vi "Recoverable Errors.vi"() -> ()   [LabVIEW 2018]
uses:
  api/Failure Information.ctl
  api/Log Record.ctl
  api/logger_class/Internal Log Levels.ctl
  api/Log Levels.ctl
  api/configuration/handlers/file_handler/File Handler.lvclass
  C:/Users/Colin/Documents/software_projects/glog/src/api/extension/formatting_handler_interface/Formatting Handler.lvclass
  custom_classes/test_handler/Test Handler.lvclass
  <vilib>/ErrorRing/Error Ring.xnode
  api/logger_class/Logger.lvclass
  api/GLog.lvlib
  <vilib>/addons/_JKI.lib/Serialization/JSON/JKI JSON Serialization.lvlib
panel:
  out "failure info":T1 {"Log Record"."timestamp" format="%<%x %.3X>T"}
  out "error out":errorcluster
  out "result":bool
  # "Locals"
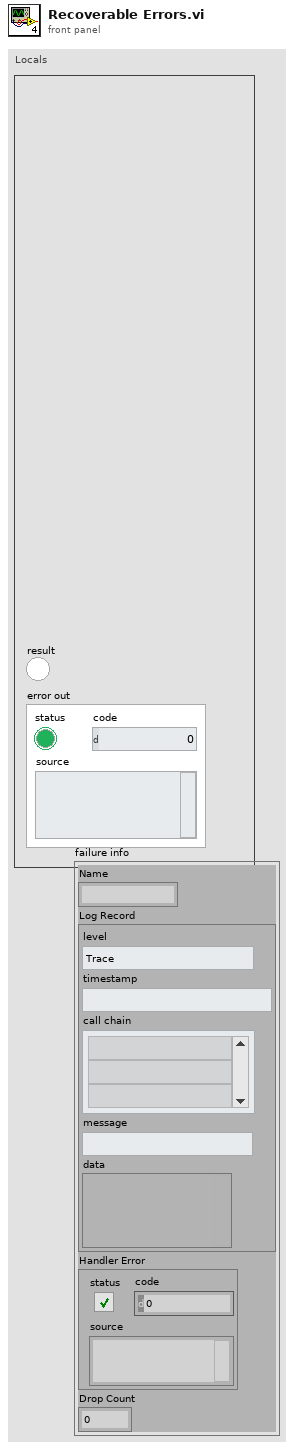
[diagram p1: front panel]
types:
  T1 = typedef "GLog.lvlib/Failure Information.ctl" = cluster{"Name":string, "Log Record":T2, "Handler Error":errorcluster, "Drop Count":u32}
  T2 = typedef "GLog.lvlib/Log Record.ctl" = cluster{"level":T3, "timestamp":timestamp, "call chain":string[], "message":string, "data":variant}
  T3 = typedef "GLog.lvlib/Internal Log Levels.ctl" = enum16{"Trace", "Debug", "Info", "Warning", "Error", "Critical", "Internal"}
  T4 = typedef "GLog.lvlib/Log Levels.ctl" = enum16{"Trace", "Debug", "Info", "Warning", "Error", "Critical"}
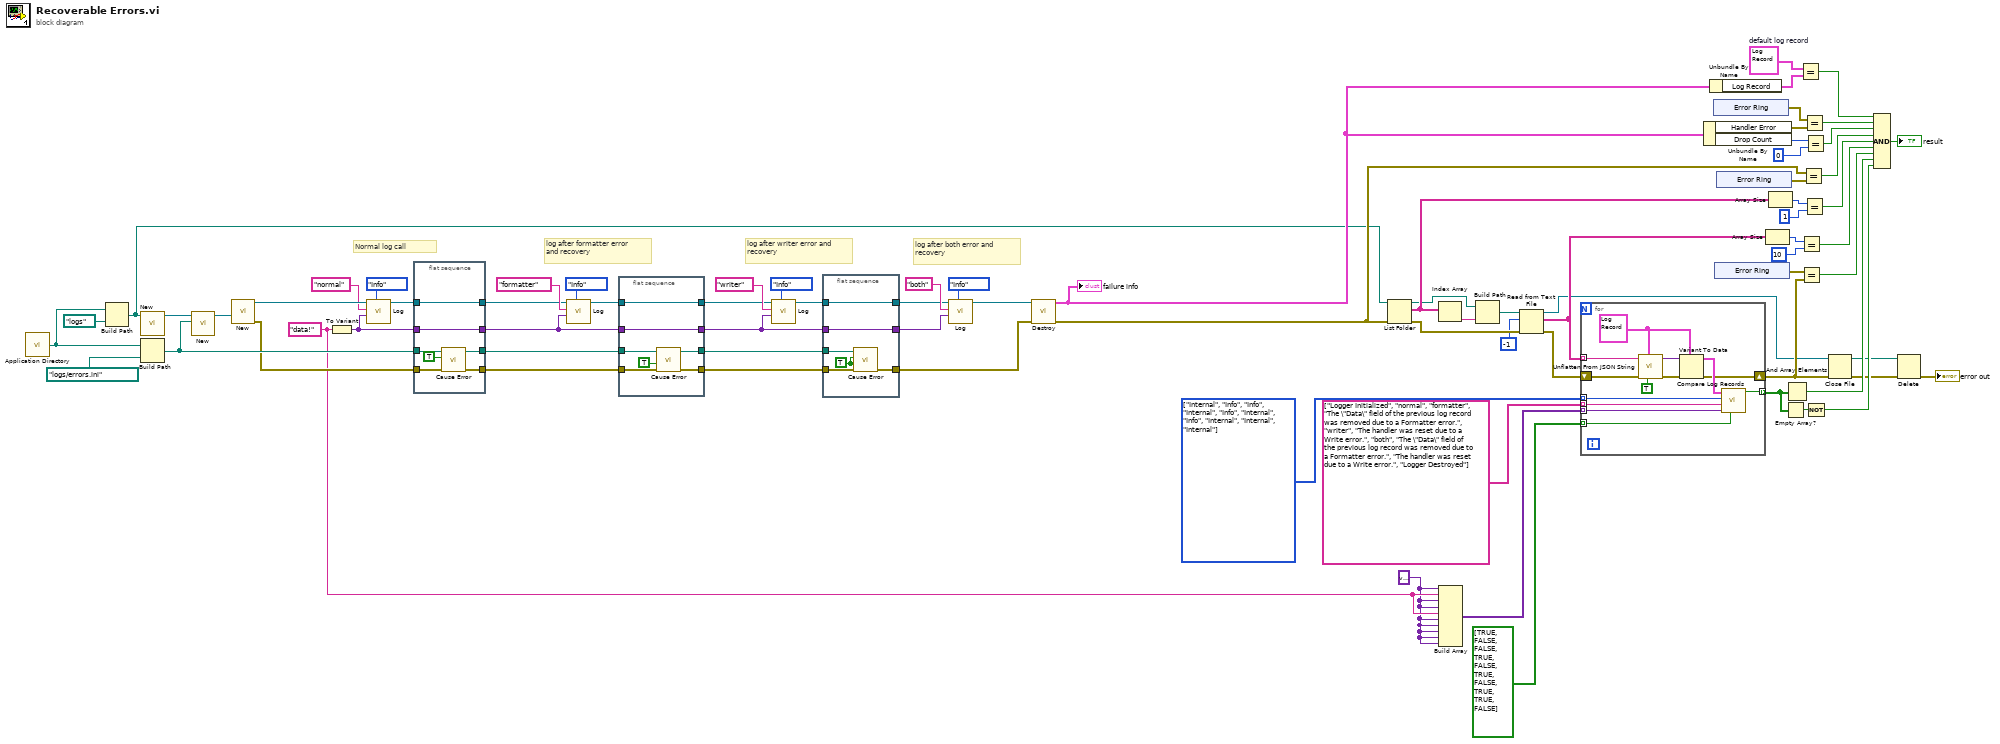
[diagram p0: block diagram]
diagram:
  w2 = variant
  w18 = T3[] [enum."Internal", enum."Info", enum."Info", enum."Internal", enum."Info", enum."Internal", enum."Info", enum."Internal", enum."Internal", enum."Internal"] items=["Trace", "Debug", "Info", "Warning", "Error", "Critical", "Internal"] ("expected log level")
  w38 = T2 {"level"=enum."Trace", "timestamp"=timestamp(0 s since 1904-01-01), "call chain"=[], "message"="", "data"=variant}  # default log record
  w15 = "data!" ("message")
  # "log after both error and recovery"
  # "log after writer error and recovery"
  # "log after formatter error and recovery"
  # "Normal log call"
  n1 = call <vilib>:"Application Directory.vi"() -> ("Application Directory"=w36:path)
  n2 = Build Path(base path=w36, name or relative path=path "logs") -> (appended path=w33:path)
  n3 = call "New.vi"("log directory (<app dir>/logs)"=w33) -> ("file handler"=w78:refnum<class "File Handler.lvclass">)  [unwired: 10 in]
  n4 = Build Path(base path=w36, name or relative path=path "logs/errors.ini") -> (appended path=w66:path)
  n5 = call "New.vi"("config file"=w66, "subhandler"=w78) -> ("test handler out"=w77:refnum<class "Test Handler.lvclass">)  [unwired: 9 in]
  n6 = call "New.vi"("log handler (file handler)"=w77) -> ("error out"=w65:errorcluster, "logger"=w75:refnum<class "Logger.lvclass">)  [unwired: 9 in]
  n7 = To Variant(anything=w15) -> (Variant=w52:variant)
  n8 = call "Log.vi"("log level"=Log_Levels."Info" ("level"), "data (null)"=w52, "message"="normal", "logger in"=w75) -> ("logger out"=w59:refnum<class "Logger.lvclass">)  [unwired: 7 in]
  n9 = flat-sequence {
    tunnel: w66 -> [w85]
    tunnel: w65 -> [w84]
    tunnel: [w83] -> w64
    tunnel: [w82] -> w63
    tunnel: [w80] -> w60
    tunnel: w59 -> [w80]
    tunnel: [w79] -> w51
    tunnel: w52 -> [w79]
    frame #0 {
      n10 = call "Cause Error.vi"("error in (no error)"=w84, "formatter error? (F)"=TRUE, "ini file path"=w85) -> ("error out"=w83:errorcluster, "ini file path"=w82:path)  [unwired: 7 in]
    }
  }
  n11 = call "Log.vi"("log level"=Log_Levels."Info" ("level"), "data (null)"=w51, "message"="formatter", "logger in"=w60) -> ("logger out"=w57:refnum<class "Logger.lvclass">)  [unwired: 7 in]
  n12 = flat-sequence {
    tunnel: w64 -> [w92]
    tunnel: w63 -> [w91]
    tunnel: [w89] -> w62
    tunnel: [w88] -> w61
    tunnel: [w87] -> w58
    tunnel: w57 -> [w87]
    tunnel: [w86] -> w49
    tunnel: w51 -> [w86]
    frame #0 {
      n13 = call "Cause Error.vi"("error in (no error)"=w92, "writer error? (F)"=TRUE, "ini file path"=w91) -> ("error out"=w88:errorcluster, "ini file path"=w89:path)  [unwired: 7 in]
    }
  }
  n14 = call "Log.vi"("log level"=Log_Levels."Info" ("level"), "data (null)"=w49, "message"="writer", "logger in"=w58) -> ("logger out"=w55:refnum<class "Logger.lvclass">)  [unwired: 7 in]
  n15 = flat-sequence {
    tunnel: w62 -> [w97]
    tunnel: w61 -> [w96]
    tunnel: [w95] -> w56
    tunnel: w55 -> [w95]
    tunnel: [w94] -> w53
    tunnel: [w93] -> w50
    tunnel: w49 -> [w93]
    frame #0 {
      w98 = TRUE ("writer error? (F)")
      n16 = call "Cause Error.vi"("error in (no error)"=w96, "writer error? (F)"=w98, "formatter error? (F)"=w98, "ini file path"=w97) -> ("error out"=w94:errorcluster)  [unwired: 6 in, 1 out]
    }
  }
  n17 = call "Log.vi"("log level"=Log_Levels."Info" ("level"), "data (null)"=w50, "message"="both", "logger in"=w56) -> ("logger out"=w54:refnum<class "Logger.lvclass">)  [unwired: 7 in]
  n18 = call "Destroy.vi"("error in (no error)"=w53, "logger in"=w54) -> ("error out"=w34:errorcluster, "failure info"=w40:T1)  [unwired: 8 in]
  "failure info" <- w40
  n19 = List Folder(path=w33, error in=w34) -> (path out=w27:path, filenames=w29:string[], error out=w25:errorcluster)  [unwired: 2 in, 1 out]
  n20 = Index Array(array=w29) -> (element=w28:string)  [unwired: 1 in]
  n21 = Build Array(w2, w15, w2, w2, w15, w2, w2, w2, w2, w2) -> (w16:variant[])
  n22 = Build Path(base path=w27, name or relative path=w28) -> (appended path=w26:path)
  n23 = Read from Text File(file (use dialog)=w26, count=-1, error in=w25) -> (refnum out=w6:refnum<file>, text=w20:string[], error out=w19:errorcluster)  [unwired: 1 in, 1 out]
  n24 = for {
    tunnel: w20 -> [w111] mode=indexing
    shift-right: [w106] -> w7
    shift-left: w19 -> [w108]
    tunnel: w18 -> [w105] mode=indexing
    tunnel: string[] ["Logger Initialized", "normal", "formatter", "The \"Data\" field of the previous log record was removed due to a Formatter error.", "writer", "The handler was reset due to a Write error.", "both", "The \"Data\" field of the previous log record was removed due to a Formatter error.", "The handler was reset due to a Write error.", "Logger Destroyed"] ("expected message") -> [w104] mode=indexing
    tunnel: w16 -> [w103] mode=indexing
    tunnel: bool[] [TRUE, FALSE, FALSE, TRUE, FALSE, TRUE, FALSE, TRUE, TRUE, FALSE] ("appended array") -> [w102] mode=indexing
    tunnel: [w101] -> w13 mode=indexing
    w100 = T2 {"level"=enum."Trace", "timestamp"=timestamp(0 s since 1904-01-01), "call chain"=[], "message"="", "data"=variant} ("default log record")
    n25 = call <vilib>:"Unflatten From JSON String.vi"("Nulls as Defaults (F)"=TRUE, "Type and Defaults"=w100, "error in (no error)"=w108, "JSON String"=w111) -> ("error out"=w110:errorcluster, "Variant"=w109:variant)  [unwired: 6 in]
    n26 = Variant To Data(error in=w110, type=w100, Variant=w109) -> (data=w107:T2, error out=w106:errorcluster)
    n27 = call "Compare Log Records.vi"("ignore data? (F)"=w102, "expected data"=w103, "expected message"=w104, "expected log level"=w105, "log record"=w107) -> ("match?"=w101:bool)  [unwired: 6 in]
  }
  n28 = Unbundle By Name(w40) -> ("Handler Error"=w48:errorcluster, "Drop Count"=w46:u32)
  n29 = Unbundle By Name(w40) -> ("Log Record"=w39:T2)
  n30 = xnode "Error Ring"() -> ("error out"=w47:errorcluster)
  n31 = xnode "Error Ring"() -> ("error out"=w14:errorcluster)
  n32 = xnode "Error Ring"() -> ("error out"=w44:errorcluster)
  n33 = Array Size(array=w20) -> (size(s)=w22:i32)
  n34 = Array Size(array=w29) -> (size(s)=w32:i32)
  n35 = Empty Array?(array=w13) -> (empty?=w12:bool)
  n36 = And Array Elements(Boolean array=w13) -> (logical AND=w10:bool)
  n37 = Equal?(x=w38, y=w39) -> (x = y?=w37:bool)
  n38 = Equal?(x=w22, y=10) -> (x = y?=w21:bool)
  n39 = Equal?(x=w14, y=w7) -> (x = y?=w11:bool)
  n40 = Equal?(x=w34, y=w44) -> (x = y?=w41:bool)
  n41 = Equal?(x=w47, y=w48) -> (x = y?=w43:bool)
  n42 = Equal?(x=w32, y=1) -> (x = y?=w30:bool)
  n43 = Equal?(x=w46, y=u32 0) -> (x = y?=w42:bool)
  n44 = Not(x=w12) -> (.not. x?=w9:bool)
  n45 = Close File(refnum=w6, error in=w7) -> (path=w5:path, error out=w4:errorcluster)
  n46 = Compound Arithmetic op=AND(w37, w43, w42, w41, w30, w21, w11, w10, w9) -> (→"result":bool)
  n47 = Delete(path (use dialog)=w5, error in=w4) -> (error out=→"error out":errorcluster)  [unwired: 3 in, 2 out]
